vi "Get Sounds.vi"(8 "error in (no error)":errorcluster, 11 "Sound":T1(ring)) -> (0 "error out":errorcluster, 3 "Sound Out":waveform(dbl))   [LabVIEW 2018]
uses:
  KorokSounds.ctl
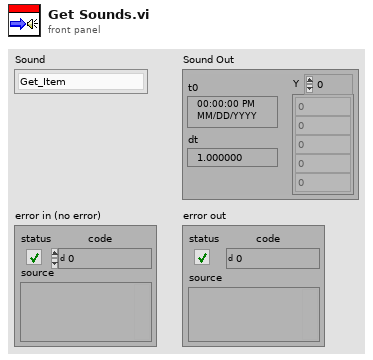
[diagram p1: front panel]
types:
  T1 = enum16{"Get_Item", "Yahaha!", "Korok_Pop", "Korok_Solve"}
  T2 = typedef "KorokSounds.ctl" = cluster{"Get_Item":waveform(dbl), "Yahaha!":waveform(dbl), "Korok_Pop":waveform(dbl), "Korok_Solve":waveform(dbl)}
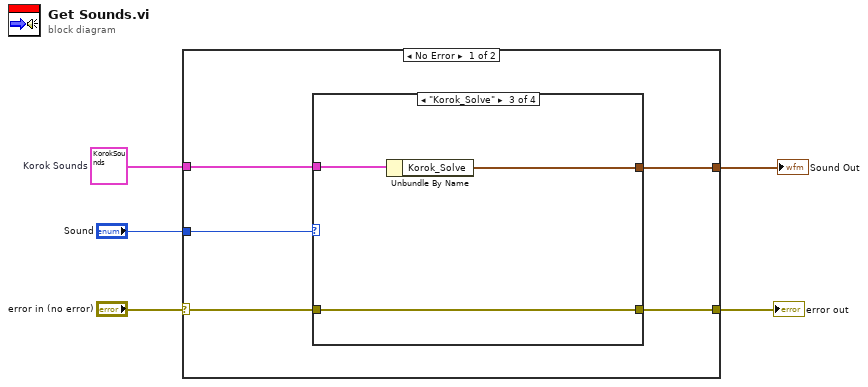
[diagram p0: block diagram]
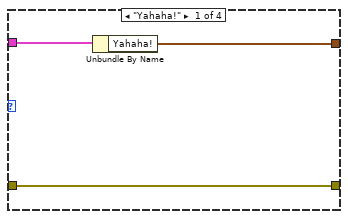
[diagram p2: hidden frame]
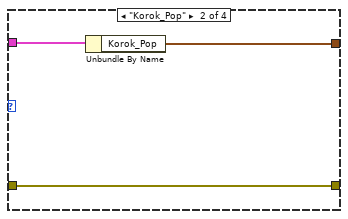
[diagram p3: hidden frame]
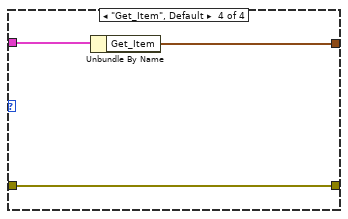
[diagram p4: hidden frame]
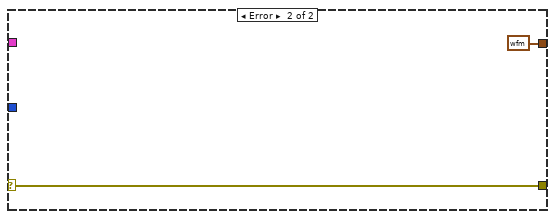
[diagram p5: hidden frame]
diagram:
  w2 = T2 {"Get_Item"={"t0"=timestamp(0 s since 1904-01-01), "dt"=2.2675736961451248e-05, "Y"=array[79488 elements]}, "Yahaha!"={"t0"=timestamp(0 s since 1904-01-01), "dt"=2.2675736961451248e-05, "Y"=array[63360 elements]}, "Korok_Pop"={"t0"=timestamp(0 s since 1904-01-01), "dt"=2.2675736961451248e-05, "Y"=array[78441 elements]}, "Korok_Solve"={"t0"=timestamp(0 s since 1904-01-01), "dt"=2.2675736961451248e-05, "Y"=array[88576 elements]}}  # Korok Sounds
  n1 = case shown="No Error" "error in (no error)" {
    selector: "error in (no error)" -> [w8 w24]
    tunnel: [w7 w24] -> w4
    tunnel: "Sound" -> [w10 _]
    tunnel: w2 -> [w9 _]
    tunnel: [w6 waveform(dbl) {"t0"=timestamp(0 s since 1904-01-01), "dt"=1.0, "Y"=[]} ("Get_Item")] -> w1
    frame No Error {
      n2 = case shown="\"Korok_Solve\"" w10 {
        tunnel: w9 -> [w12 w15 w18 w21]
        tunnel: w8 -> [w13 w16 w19 w22]
        tunnel: [w13 w16 w19 w22] -> w7
        tunnel: [w11 w14 w17 w20] -> w6
        frame "Yahaha!" {
          n3 = Unbundle By Name(w12) -> ("Yahaha!"=w11:waveform(dbl))
        }
        frame "Korok_Pop" {
          n4 = Unbundle By Name(w15) -> ("Korok_Pop"=w14:waveform(dbl))
        }
        frame "Korok_Solve" {
          n5 = Unbundle By Name(w18) -> ("Korok_Solve"=w17:waveform(dbl))
        }
        frame "Get_Item", Default {
          n6 = Unbundle By Name(w21) -> ("Get_Item"=w20:waveform(dbl))
        }
      }
    }
    frame Error {
    }
  }
  "error out" <- w4
  "Sound Out" <- w1
